vi "File.Simple Text Logger.vi"(5 "AddDateTimeStamp":bool=TRUE, 7 "Folder":path=path "c:/MTE/Logs", 10 "Data":string, 11 "Name(LessExt)":string="Data Log") -> ()   [LabVIEW 2019]
uses:
  <vilib>/KATE/Files/File Utils.lvlib
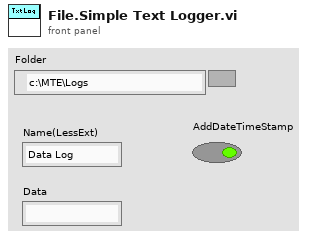
[diagram p1: front panel]
types:
  T1 = enum16{"open", "replace", "create", "open or create", "replace or create", "replace or create with confirmation"}
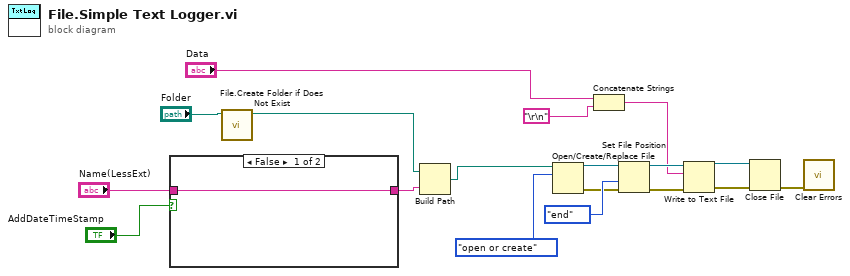
[diagram p0: block diagram]
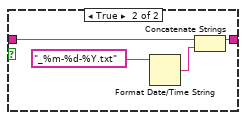
[diagram p2: hidden frame]
diagram:
  n1 = case shown="False" "AddDateTimeStamp" {
    tunnel: "Name(LessExt)" -> [w19 w21]
    tunnel: [w19 w20] -> w12
    frame False {
    }
    frame True {
      n2 = Format Date/Time String(time format string (%c)="_%m-%d-%Y.txt") -> (date/time string=w22:string)  [unwired: 2 in]
      n3 = Concatenate Strings(w21, w22) -> (w20:string)
    }
  }
  n4 = call <vilib>:"File.Create Folder if Does Not Exist.vi"("Path"="Folder") -> ("Dup Path"=w13:path)  [unwired: 8 in, 2 out]
  n5 = Build Path(base path=w13, name or relative path=w12) -> (appended path=w11:path)
  n6 = Open/Create/Replace File(file path (use dialog)=w11, operation (0:open)=T1."open or create") -> (refnum out=w17:refnum<file>, error out=w16:errorcluster)  [unwired: 4 in, 1 out]
  n7 = Concatenate Strings("Data", "\r\n") -> (w1:string)
  n8 = Set File Position(refnum=w17, from (0:start)=enum16{"start", "end", "current"}."end", error in=w16) -> (refnum out=w9:refnum<file>, error out=w8:errorcluster)  [unwired: 1 in]
  n9 = Write to Text File(file (use dialog)=w9, text=w1, error in=w8) -> (refnum out=w6:refnum<file>, error out=w7:errorcluster)  [unwired: 1 in, 1 out]
  n10 = Close File(refnum=w6, error in=w7) -> (error out=w5:errorcluster)  [unwired: 1 out]
  n11 = call <vilib>:"Clear Errors.vi"("error in (no error)"=w5) -> ()  [unwired: 5 in, 2 out]
